vi "Práctica01_Ejercicio1_2.vi"() -> ()   [LabVIEW 2020]
panel:
  in  "Boolean":bool
  out "Numeric 2":i32
  out "Numeric":i32
  in  "Materias a cursar este semestre":u8(slide) scale=0.0..100.0
  in  "Salir de la Universidad":bool
  in  "Cantidad de Semestres Faltantes":dbl(knob) scale=0.0..10.0
  out "Años que faltan por cursar":dbl(knob) scale=0.0..10.0
  out "No":bool
  in  "¿Le sabes al LAB VIEW?":bool
  out "Alumno(a)":string
  out "ETS's a presentar":u8(slide) scale=0.0..100.0
  in  "Alumno(a)":string
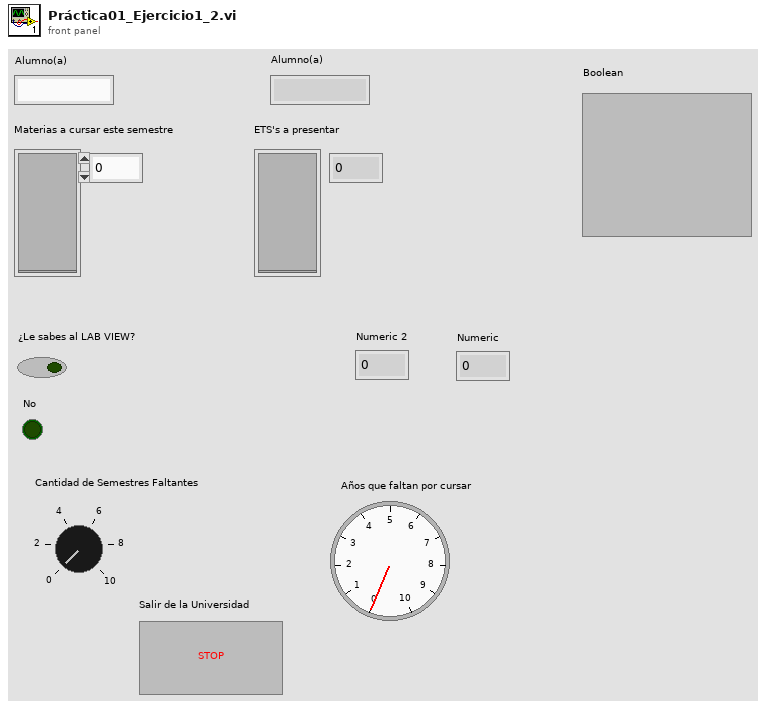
[diagram p1: front panel]
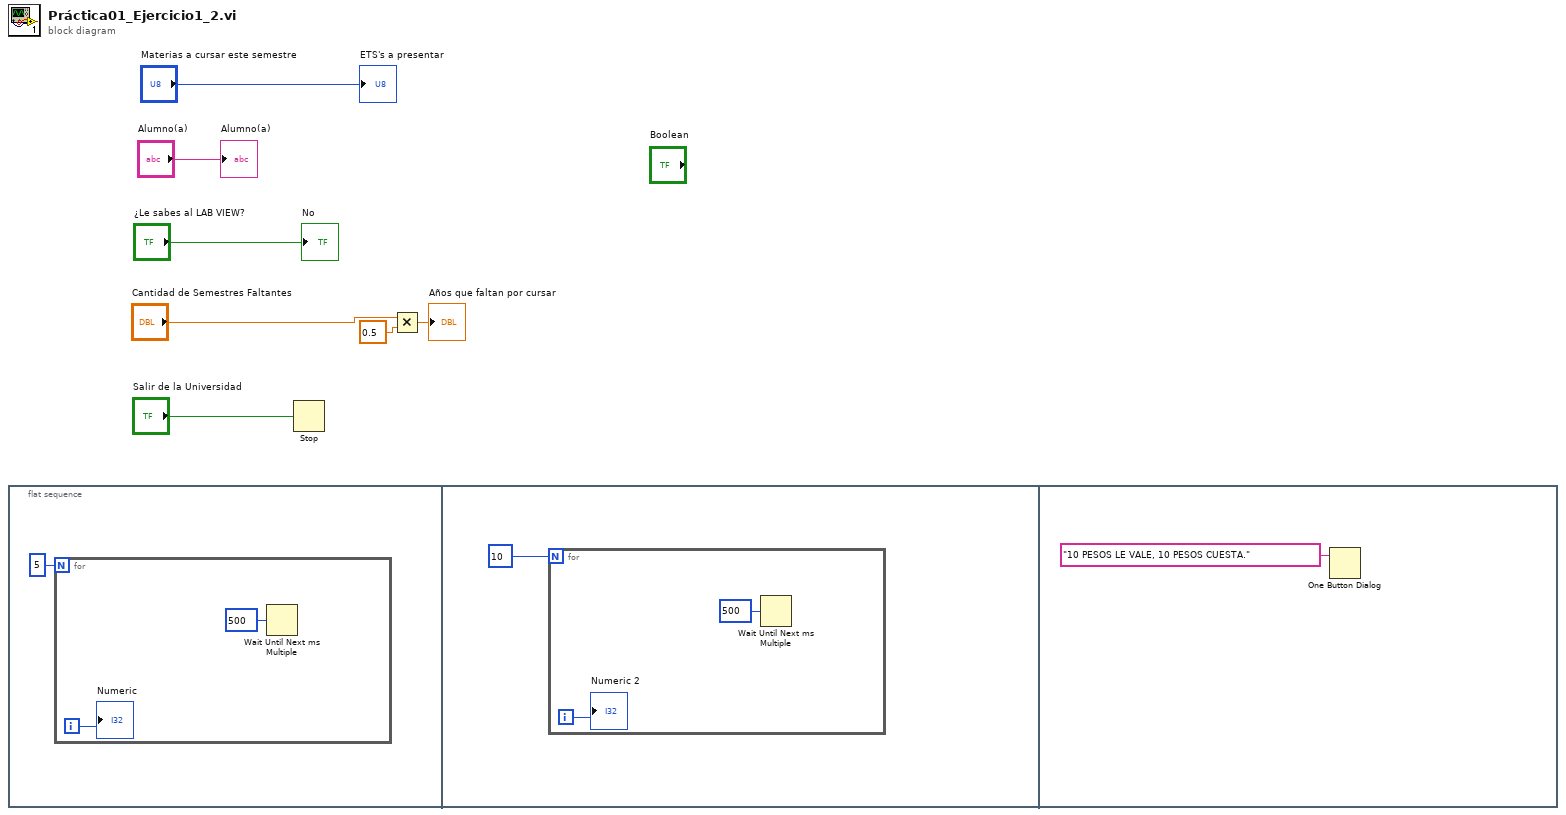
[diagram p0: block diagram]
diagram:
  n1 = flat-sequence {
    frame #0 {
      n2 = for {
        N: 5 -> [_]
        i -> [w10]
        n3 = Wait Until Next ms Multiple(millisecond multiple=u32 500) -> ()  [unwired: 1 out]
        "Numeric" <- w10
      }
    }
    frame #1 {
      n4 = for {
        N: 10 -> [_]
        i -> [w13]
        n5 = Wait Until Next ms Multiple(millisecond multiple=u32 500) -> ()  [unwired: 1 out]
        "Numeric 2" <- w13
      }
    }
    frame #2 {
      n6 = One Button Dialog(message="10 PESOS LE VALE, 10 PESOS CUESTA.") -> ()  [unwired: 1 in, 1 out]
    }
  }
  n7 = Stop(stop? (T)="Salir de la Universidad") -> ()
  n8 = Multiply(x="Cantidad de Semestres Faltantes", y=0.5) -> (x*y=→"Años que faltan por cursar":dbl)
  "ETS's a presentar" <- "Materias a cursar este semestre"
  "Alumno(a)" <- "Alumno(a)"
  "No" <- "¿Le sabes al LAB VIEW?"
